vi "To String.vi"(8 "error in (no error)":errorcluster, 11 "U32 Array in":refnum<class "U32 Array.lvclass">) -> (0 "error out":errorcluster, 2 "String":string)   [LabVIEW 2020, in "Data.lvlib" / "U32 Array.lvclass"]
doc: "Convert 'Generic Data in' to a string."
uses:
  U32 Array.lvclass
  U32 Array.lvclass/U32 Array.ctl
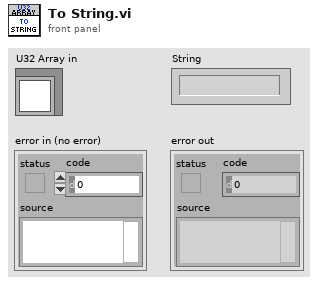
[diagram p1: front panel]
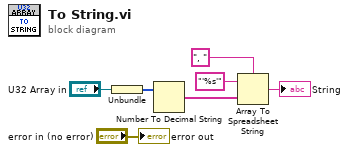
[diagram p0: block diagram]
diagram:
  n1 = Unbundle("U32 Array in") -> (w2:u32[])
  n2 = Number To Decimal String(number=w2) -> (decimal integer string=w1:string[])  [unwired: 1 in]
  n3 = Array To Spreadsheet String(delimiter (Tab)=", ", array=w1, 3:"'%s'" ("format string")) -> (spreadsheet string=→"String":string)
  "error out" <- "error in (no error)"
